vi "ep_Detect Signaling Voltage Telegram.vi"(0 "signaling voltage RMS [V]":dbl, 1 "phase":T1, 2 "restart? (F)":bool, 5 "signaling current RMS [A]":dbl, 7 "detected signaling frequency [Hz]":dbl, 9 "nominal voltage [V]":dbl=230.0, 11 "signaling voltage event settings":T2={"signaling detection threshold [%]"=0.3, "signaling starting log. 1 length (T1) [sec]"=2.99, "signaling starting log. 0 length (T2) [sec]"=2.33, "signaling message max. length [sec]"=64.0}, 12 "time stamp":timestamp, 13 "interval length [sec]":dbl, 14 "error in (no error)":errorcluster) -> (4 "Telegram":T3={"event time"=timestamp(0 s since 1904-01-01), "phase"=enum."Phase A (L1)", "signaling frequency [Hz]"=0.0, "event voltage max. [V]"=0.0, "event voltage log. 1 [V]"=0.0, "event voltage log. 0 [V]"=0.0, "event current max. [A]"=0.0, "event current log. 1 [A]"=0.0, "event current log. 0 [A]"=0.0, "event digital waveform"={"t0"=timestamp(0 s since 1904-01-01), "dt"=1.0, "Y"={"transitions"=[], "data"=[]}}}, 6 "data valid?":bool, 15 "error out":errorcluster)   [LabVIEW 2014, in "NI_EP_Power Quality.lvlib"]
uses:
  <vilib>/addons/Electrical Power/PQ/NI_EP_Power Quality.lvlib
  <vilib>/addons/Electrical Power/PQ/Common/Controls/ep_Phase.ctl
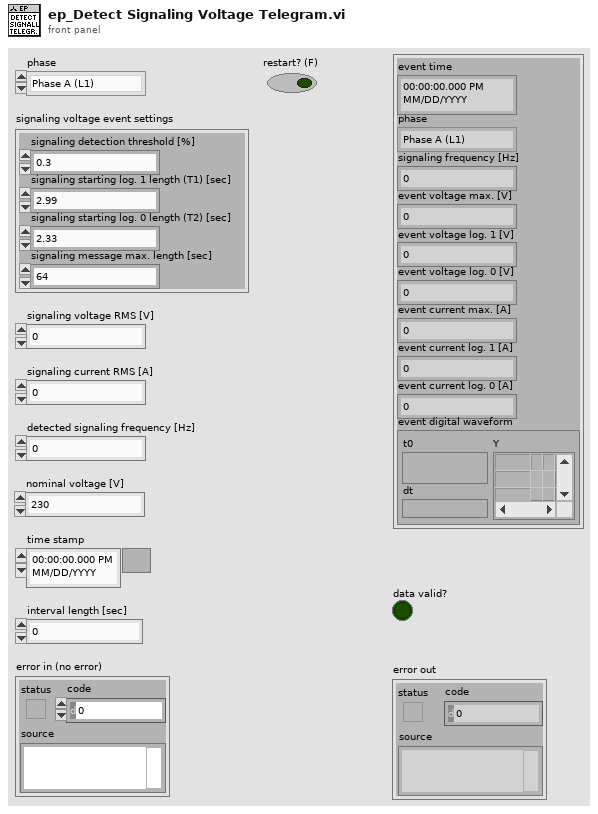
[diagram p1: front panel]
types:
  T1 = typedef "NI_EP_Power Quality.lvlib/ep_Phase.ctl" = enum16{"Phase A (L1)", "Phase B (L2)", "Phase C (L3)", "Phase N", "~3 Phases"}
  T2 = cluster{"signaling detection threshold [%]":dbl, "signaling starting log. 1 length (T1) [sec]":dbl, "signaling starting log. 0 length (T2) [sec]":dbl, "signaling message max. length [sec]":dbl}
  T3 = cluster{"event time":timestamp, "phase":T1, "signaling frequency [Hz]":dbl, "event voltage max. [V]":dbl, "event voltage log. 1 [V]":dbl, "event voltage log. 0 [V]":dbl, "event current max. [A]":dbl, "event current log. 1 [A]":dbl, "event current log. 0 [A]":dbl, "event digital waveform":digitalwaveform}
  T4 = cluster{"event time":timestamp, "phase":T1, "signaling frequency":dbl, "event voltage max.":dbl, "event voltage log. 1":dbl, "event voltage log. 0":dbl, "event current max.":dbl, "event current log. 1":dbl, "event current log. 0":dbl, "event digital waveform":digitalwaveform}
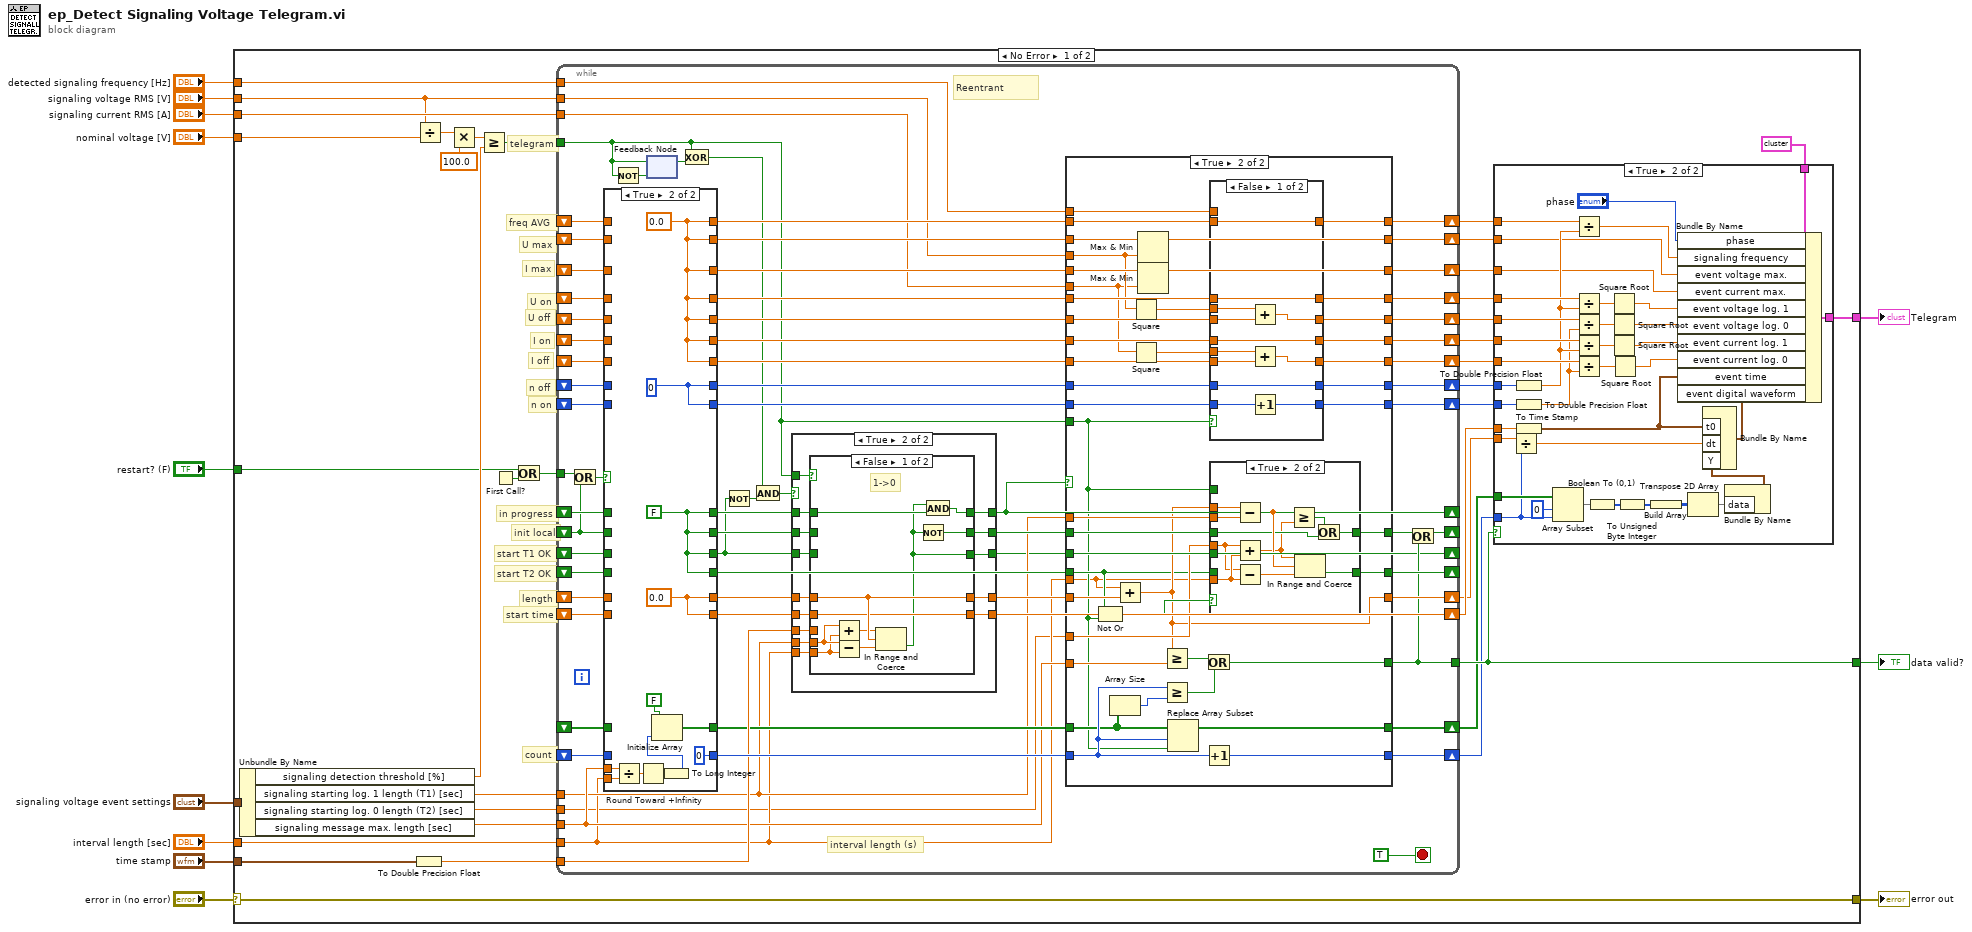
[diagram p0: block diagram]
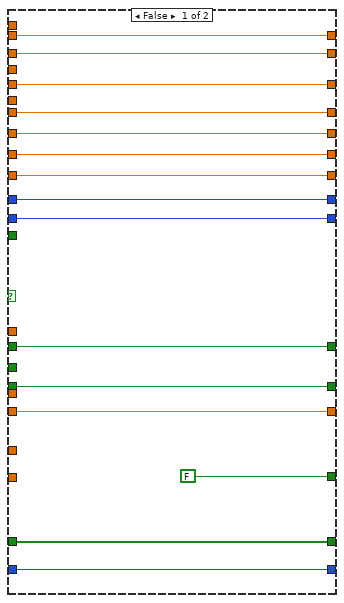
[diagram p3: hidden frame]
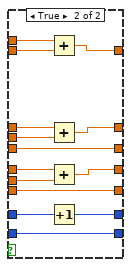
[diagram p4: hidden frame]
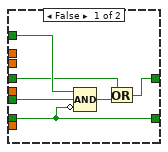
[diagram p5: hidden frame]
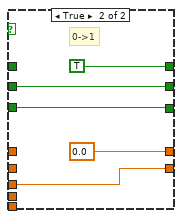
[diagram p7: hidden frame]
diagram:
  n1 = case shown="No Error" "error in (no error)" {
    selector: "error in (no error)" -> [w13 w324]
    tunnel: "signaling voltage event settings" -> [w48 _]
    tunnel: "time stamp" -> [w47 _]
    tunnel: "signaling current RMS [A]" -> [w45 _]
    tunnel: "detected signaling frequency [Hz]" -> [w44 _]
    tunnel: "interval length [sec]" -> [w42 _]
    tunnel: "nominal voltage [V]" -> [w38 _]
    tunnel: "signaling voltage RMS [V]" -> [w34 _]
    tunnel: [w23 _] -> w5
    tunnel: [w19 _] -> w4
    tunnel: "restart? (F)" -> [w14 _]
    tunnel: [w13 w324] -> w1
    frame No Error {
      # "start time"
      # "freq AVG"
      # "I max"
      # "U max"
      # "U on"
      # "U off"
      # "I off"
      # "I on"
      # "n off"
      # "n on"
      # "telegram"
      # "count"
      # "length"
      # "start T2 OK"
      # "start T1 OK"
      # "init local"
      # "in progress"
      n2 = Unbundle By Name(w48) -> ("signaling detection threshold [%]"=w36:dbl, "signaling starting log. 1 length (T1) [sec]"=w43:dbl, "signaling starting log. 0 length (T2) [sec]"=w20:dbl, "signaling message max. length [sec]"=w37:dbl)
      n3 = To Double Precision Float(number=w47) -> (double precision float=w46:dbl)
      n4 = Divide(x=w34, y=w38) -> (x/y=w40:dbl)
      n5 = Multiply(x=w40, y=100.0) -> (x*y=w39:dbl)
      n6 = Greater Or Equal?(x=w39, y=w36) -> (x >= y?=w35:bool)
      n7 = First Call?() -> (First Call?: T/F=w16:bool)
      n8 = Or(x=w14, y=w16) -> (x .or. y?=w15:bool)
      n9 = while {
        shift-left: _ -> [w120]
        shift-right: [w101] -> w33
        shift-left: _ -> [w122]
        shift-right: [w103] -> w32
        shift-left: _ -> [w124]
        shift-right: [w102] -> w31
        shift-left: _ -> [w126]
        shift-right: [w99] -> w30
        shift-left: _ -> [w128]
        shift-right: [w98] -> w29
        shift-left: _ -> [w130]
        shift-right: [w97] -> w28
        shift-left: _ -> [w132]
        shift-right: [w95] -> w27
        shift-left: _ -> [w135]
        shift-right: [w96] -> w26
        shift-left: _ -> [w136]
        shift-right: [w100] -> w25
        shift-left: _ -> [w144]
        shift-right: [w142] -> w18
        shift-left: _ -> [w147]
        shift-right: [w141] -> w17
        shift-left: _ -> [w149]
        shift-right: [w148] -> _
        shift-left: _ -> [w150]
        shift-right: [w87] -> _
        tunnel: w15 -> [w155]
        shift-left: _ -> [w105]
        shift-right: [w88] -> _
        shift-left: _ -> [w158]
        shift-right: [w152] -> _
        tunnel: [w93] -> w23
        tunnel: w46 -> [w118]
        tunnel: w42 -> [w90]
        tunnel: w34 -> [w117]
        tunnel: w45 -> [w116]
        tunnel: w44 -> [w115]
        tunnel: w43 -> [w91]
        tunnel: w37 -> [w92]
        shift-right: [w112] -> w22
        shift-left: _ -> [w114]
        shift-right: [w109] -> w24
        shift-left: _ -> [w111]
        tunnel: w35 -> [w104]
        tunnel: w20 -> [w89]
        stop <- TRUE stop-if-true
        # "interval length (s)"
        # "Reentrant"
        n10 = Or(x=w155, y=w105) -> (x .or. y?=w154:bool)
        n11 = case shown="True" w154 {
          tunnel: [w311 w320] -> w157
          tunnel: w158 -> [w311 _]
          tunnel: [w310 w320] -> w153
          tunnel: w105 -> [w310 _]
          tunnel: [w309 w320] -> w137
          tunnel: w150 -> [w309 _]
          tunnel: [w308 w320] -> w139
          tunnel: w149 -> [w308 _]
          tunnel: [w307 w313] -> w146
          tunnel: w147 -> [w307 _]
          tunnel: [w306 0 ("i")] -> w143
          tunnel: w144 -> [w306 _]
          tunnel: w136 -> [w305 _]
          tunnel: w135 -> [w304 _]
          tunnel: [w305 w321] -> w134
          tunnel: [w304 w321] -> w133
          tunnel: [w303 w322] -> w131
          tunnel: w132 -> [w303 _]
          tunnel: [w302 w322] -> w129
          tunnel: w130 -> [w302 _]
          tunnel: [w301 w322] -> w127
          tunnel: w128 -> [w301 _]
          tunnel: [w300 w322] -> w125
          tunnel: w126 -> [w300 _]
          tunnel: [w299 w322] -> w123
          tunnel: w124 -> [w299 _]
          tunnel: [w298 w322] -> w121
          tunnel: w122 -> [w298 _]
          tunnel: [w297 w322] -> w119
          tunnel: w120 -> [w297 _]
          tunnel: w92 -> [_ w317]
          tunnel: w90 -> [_ w316]
          tunnel: [w296 w314] -> w113
          tunnel: w114 -> [w296 _]
          tunnel: [w295 w313] -> w110
          tunnel: w111 -> [w295 _]
          frame False {
          }
          frame True {
            w322 = 0.0
            w321 = u32 0
            w313 = 0.0 ("Tim 1")
            w320 = FALSE ("StartOK")
            n12 = Divide(x=w317, y=w316) -> (x/y=w318:dbl)
            n13 = Round Toward +Infinity(x=w318) -> (ceil(x): smallest int >= x=w319:dbl)
            n14 = To Long Integer(number=w319) -> (32bit integer=w312:i32)
            n15 = Initialize Array(FALSE ("StartOK"), w312) -> (w314:bool[])
          }
        }
        n16 = Not(x=w104) -> (.not. x?=w108:bool)
        n17 = feedback-in #1(w104) -> ()
        n18 = feedback #1(w108) -> (w107:bool)
        n19 = Exclusive Or(1:w107, 2:w104) -> (0:w106:bool)
        n20 = Not(x=w137) -> (.not. x?=w140:bool)
        n21 = And(x=w106, y=w140) -> (x .and. y?=w138:bool)
        n22 = case shown="True" w138 {
          tunnel: [w265 w278] -> w152
          tunnel: w157 -> [w265 w279]
          tunnel: w153 -> [w264 w268]
          tunnel: [w264 w277] -> w151
          tunnel: [w263 w275] -> w87
          tunnel: w137 -> [w263 w276]
          tunnel: w146 -> [w262 w273]
          tunnel: [w262 w272] -> w145
          tunnel: w104 -> [_ w274]
          tunnel: w118 -> [_ w271]
          tunnel: [w261 w270] -> w109
          tunnel: w110 -> [w261 w269]
          tunnel: w91 -> [_ w267]
          tunnel: w90 -> [_ w266]
          frame False {
          }
          frame True {
            n23 = case shown="False" w274 {
              tunnel: [w286 TRUE ("Begin")] -> w278
              tunnel: w279 -> [w287 _]
              tunnel: [w284 w293] -> w275
              tunnel: w276 -> [_ w293]
              tunnel: w273 -> [w289 _]
              tunnel: [w289 0.0 ("Tim 1")] -> w272
              tunnel: w271 -> [_ w291]
              tunnel: [w288 w291] -> w270
              tunnel: w269 -> [w288 _]
              tunnel: [w285 w290] -> w277
              tunnel: w268 -> [_ w290]
              tunnel: w267 -> [w283 _]
              tunnel: w266 -> [w282 _]
              frame False {
                # "1->0"
                n24 = Add(x=w283, y=w282) -> (x+y=w281:dbl)
                n25 = Subtract(x=w283, y=w282) -> (x-y=w280:dbl)
                n26 = In Range and Coerce(upper limit=w281, x=w289, lower limit=w280) -> (In Range?=w284:bool)  [unwired: 1 out]
                n27 = Not(x=w284) -> (.not. x?=w285:bool)
                n28 = And(x=w284, y=w287) -> (x .and. y?=w286:bool)
              }
              frame True {
                # "0->1"
              }
            }
          }
        }
        n29 = case shown="True" w152 {
          tunnel: [FALSE w213] -> w93
          tunnel: [w172 w216] -> w94
          tunnel: w151 -> [w172 w217]
          tunnel: w139 -> [w171 w177]
          tunnel: [w171 w215] -> w148
          tunnel: w145 -> [w170 w179]
          tunnel: [w170 w178] -> w141
          tunnel: w143 -> [w169 w187]
          tunnel: [w169 w212] -> w142
          tunnel: w104 -> [_ w175]
          tunnel: w134 -> [w167 w211]
          tunnel: w133 -> [w168 w210]
          tunnel: [w168 w209] -> w96
          tunnel: [w167 w208] -> w100
          tunnel: w131 -> [w165 w207]
          tunnel: w129 -> [w164 w206]
          tunnel: w127 -> [w163 w205]
          tunnel: w125 -> [w162 w204]
          tunnel: w123 -> [w161 w197]
          tunnel: w121 -> [w160 w196]
          tunnel: w119 -> [w166 w203]
          tunnel: [w166 w202] -> w101
          tunnel: [w165 w198] -> w95
          tunnel: [w164 w199] -> w97
          tunnel: [w163 w200] -> w98
          tunnel: [w162 w201] -> w99
          tunnel: [w161 w194] -> w102
          tunnel: [w160 w195] -> w103
          tunnel: w90 -> [_ w174]
          tunnel: w117 -> [_ w191]
          tunnel: w116 -> [_ w190]
          tunnel: w115 -> [_ w189]
          tunnel: w91 -> [_ w188]
          tunnel: w113 -> [w159 w183]
          tunnel: [w159 w186] -> w112
          tunnel: w92 -> [_ w184]
          tunnel: w89 -> [_ w180]
          tunnel: w87 -> [_ w176]
          frame False {
          }
          frame True {
            n30 = Not Or(1:w175, 2:w177) -> (0:w182:bool)
            n31 = Array Size(array=w183) -> (size(s)=w185:i32)
            n32 = Add(x=w174, y=w179) -> (x+y=w178:dbl)
            n33 = Square(x=w191) -> (x^2=w193:dbl)
            n34 = Square(x=w190) -> (x^2=w192:dbl)
            n35 = Max & Min(x=w196, y=w191) -> (max(x,y)=w195:dbl)  [unwired: 1 out]
            n36 = Max & Min(x=w197, y=w190) -> (max(x,y)=w194:dbl)  [unwired: 1 out]
            n37 = Greater Or Equal?(x=w178, y=w184) -> (x >= y?=w214:bool)
            n38 = Greater Or Equal?(x=w187, y=w185) -> (x >= y?=w181:bool)
            n39 = Replace Array Subset(array=w183, new element=w175, index=w187) -> (w186:bool[])
            n40 = Or(x=w214, y=w181) -> (x .or. y?=w213:bool)
            n41 = Increment(x=w187) -> (x+1=w212:i32)
            n42 = case shown="False" w175 {
              tunnel: w189 -> [_ w238]
              tunnel: [w222 w232] -> w208
              tunnel: w211 -> [w229 w232]
              tunnel: [w221 w231] -> w209
              tunnel: w210 -> [w221 w243]
              tunnel: [w218 w242] -> w198
              tunnel: w207 -> [w219 w242]
              tunnel: [w226 w233] -> w199
              tunnel: w206 -> [w226 w236]
              tunnel: [w223 w241] -> w200
              tunnel: w205 -> [w225 w241]
              tunnel: [w227 w234] -> w201
              tunnel: w204 -> [w227 w237]
              tunnel: [w228 w239] -> w202
              tunnel: w203 -> [w228 w240]
              tunnel: w193 -> [w224 w230]
              tunnel: w192 -> [w220 w235]
              frame False {
                n43 = Add(x=w224, y=w225) -> (x+y=w223:dbl)
                n44 = Add(x=w220, y=w219) -> (x+y=w218:dbl)
                n45 = Increment(x=w229) -> (x+1=w222:u32)
              }
              frame True {
                n46 = Add(x=w238, y=w240) -> (x+y=w239:dbl)
                n47 = Add(x=w237, y=w230) -> (x+y=w234:dbl)
                n48 = Add(x=w236, y=w235) -> (x+y=w233:dbl)
                n49 = Increment(x=w243) -> (x+1=w231:u32)
              }
            }
            n50 = case shown="True" w182 {
              tunnel: w178 -> [_ w259]
              tunnel: w217 -> [w245 w253]
              tunnel: [w244 w255] -> w216
              tunnel: w177 -> [w249 _]
              tunnel: [w249 w260] -> w215
              tunnel: w188 -> [_ w257]
              tunnel: w180 -> [_ w250]
              tunnel: w174 -> [_ w254]
              tunnel: w176 -> [w248 _]
              tunnel: w175 -> [w247 _]
              frame False {
                n51 = Compound Arithmetic op=AND(w247, w248, invert w249) -> (w246:bool)
                n52 = Or(x=w245, y=w246) -> (x .or. y?=w244:bool)
              }
              frame True {
                n53 = Subtract(x=w259, y=w257) -> (x-y=w258:dbl)
                n54 = Add(x=w250, y=w254) -> (x+y=w251:dbl)
                n55 = Subtract(x=w250, y=w254) -> (x-y=w252:dbl)
                n56 = Greater Or Equal?(x=w258, y=w251) -> (x >= y?=w256:bool)
                n57 = In Range and Coerce(upper limit=w251, x=w258, lower limit=w252) -> (In Range?=w260:bool)  [unwired: 1 out]
                n58 = Or(x=w256, y=w253) -> (x .or. y?=w255:bool)
              }
            }
          }
        }
        n59 = Or(x=w94, y=w93) -> (x .or. y?=w88:bool)
      }
      n60 = case shown="True" w23 {
        tunnel: w26 -> [_ w84]
        tunnel: w25 -> [_ w85]
        tunnel: w33 -> [_ w86]
        tunnel: w32 -> [_ w70]
        tunnel: w31 -> [_ w58]
        tunnel: w30 -> [_ w83]
        tunnel: w29 -> [_ w82]
        tunnel: w28 -> [_ w81]
        tunnel: w27 -> [_ w80]
        tunnel: [w49 w73] -> w19
        tunnel: T4 {"event time"=timestamp(0 s since 1904-01-01), "phase"=enum."Phase A (L1)", "signaling frequency"=0.0, "event voltage max."=0.0, "event voltage log. 1"=0.0, "event voltage log. 0"=0.0, "event current max."=0.0, "event current log. 1"=0.0, "event current log. 0"=0.0, "event digital waveform"={"t0"=timestamp(0 s since 1904-01-01), "dt"=1.0, "Y"={"transitions"=[], "data"=[]}}} ("signaling voltage event") -> [w49 w72]
        tunnel: w22 -> [_ w56]
        tunnel: w24 -> [_ w62]
        tunnel: w18 -> [_ w52]
        tunnel: w17 -> [_ w53]
        frame False {
        }
        frame True {
          n61 = Divide(x=w53, y=w52) -> (x/y=w51:dbl)
          n62 = To Double Precision Float(number=w84) -> (double precision float=w79:dbl)
          n63 = To Double Precision Float(number=w85) -> (double precision float=w78:dbl)
          n64 = To Time Stamp(1:w62) -> (0:w60:timestamp)
          n65 = Array Subset(array=w56, index=0, length=w52) -> (w55:bool[])
          n66 = Divide(x=w86, y=w79) -> (x/y=w71:dbl)
          n67 = Divide(x=w83, y=w79) -> (x/y=w77:dbl)
          n68 = Divide(x=w82, y=w78) -> (x/y=w76:dbl)
          n69 = Divide(x=w81, y=w79) -> (x/y=w75:dbl)
          n70 = Divide(x=w80, y=w78) -> (x/y=w74:dbl)
          n71 = Boolean To (0,1)(Boolean=w55) -> (0, 1=w64:i16[])
          n72 = Square Root(x=w77) -> (sqrt(x)=w59:dbl)
          n73 = Square Root(x=w76) -> (sqrt(x)=w69:dbl)
          n74 = Square Root(x=w75) -> (sqrt(x)=w68:dbl)
          n75 = Square Root(x=w74) -> (sqrt(x)=w67:dbl)
          n76 = To Unsigned Byte Integer(number=w64) -> (unsigned 8bit integer=w66:u8[])
          n77 = Build Array(w66) -> (w65:u8[][])
          n78 = Transpose 2D Array(2D array=w65) -> (transposed array=w63:u8[][])
          n79 = Bundle By Name("data"=w63) -> (w50:digitaldata)  [unwired: 1 in]
          n80 = Bundle By Name("t0"=w60, "dt"=w51, "Y"=w50) -> (w57:digitalwaveform)  [unwired: 1 in]
          n81 = Bundle By Name(cluster=w72, "phase"="phase", "signaling frequency"=w71, "event voltage max."=w70, "event current max."=w58, "event voltage log. 1"=w59, "event voltage log. 0"=w69, "event current log. 1"=w68, "event current log. 0"=w67, "event time"=w60, "event digital waveform"=w57) -> (w73:T4)
        }
      }
    }
    frame Error {
    }
  }
  "Telegram" <- w4
  "data valid?" <- w5
  "error out" <- w1
